vi "b-field one sensor.vi"(0 "magnet location params":T1, 5 "x sensor":dbl, 6 "y sensor":dbl, 7 "z sensor":dbl) -> (20 "Bx (uT)":dbl, 21 "By (uT)":dbl, 22 "Bz (uT)":dbl, 25 "dBx":dbl[](array[numeric]), 26 "dBy":dbl[](array[numeric]), 27 "dBz":dbl[](array[numeric]))   [LabVIEW 2017]
uses:
  typedefs/magnet location fit result.ctl
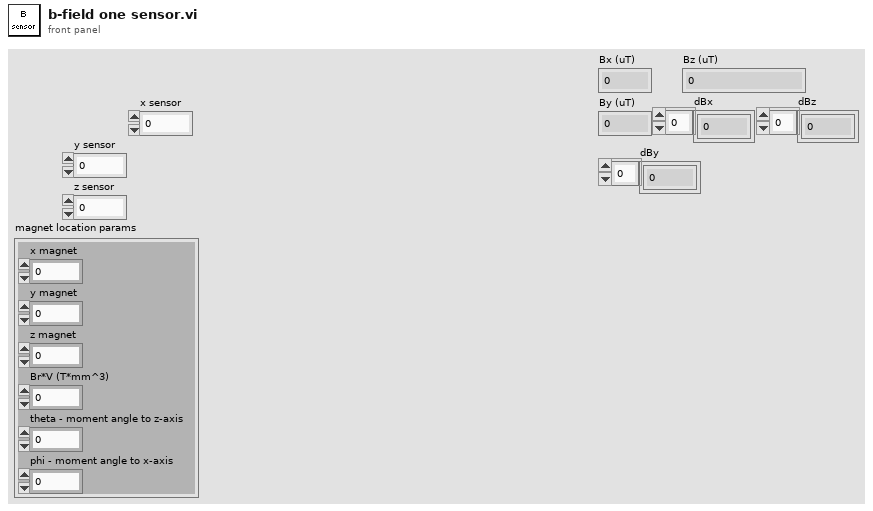
[diagram p1: front panel]
types:
  T1 = typedef "magnet location fit result.ctl" = cluster{"x magnet":dbl, "y magnet":dbl, "z magnet":dbl, "Br*V (T*mm^3)":dbl, "theta - moment angle to z-axis":dbl, "phi - moment angle to x-axis":dbl}
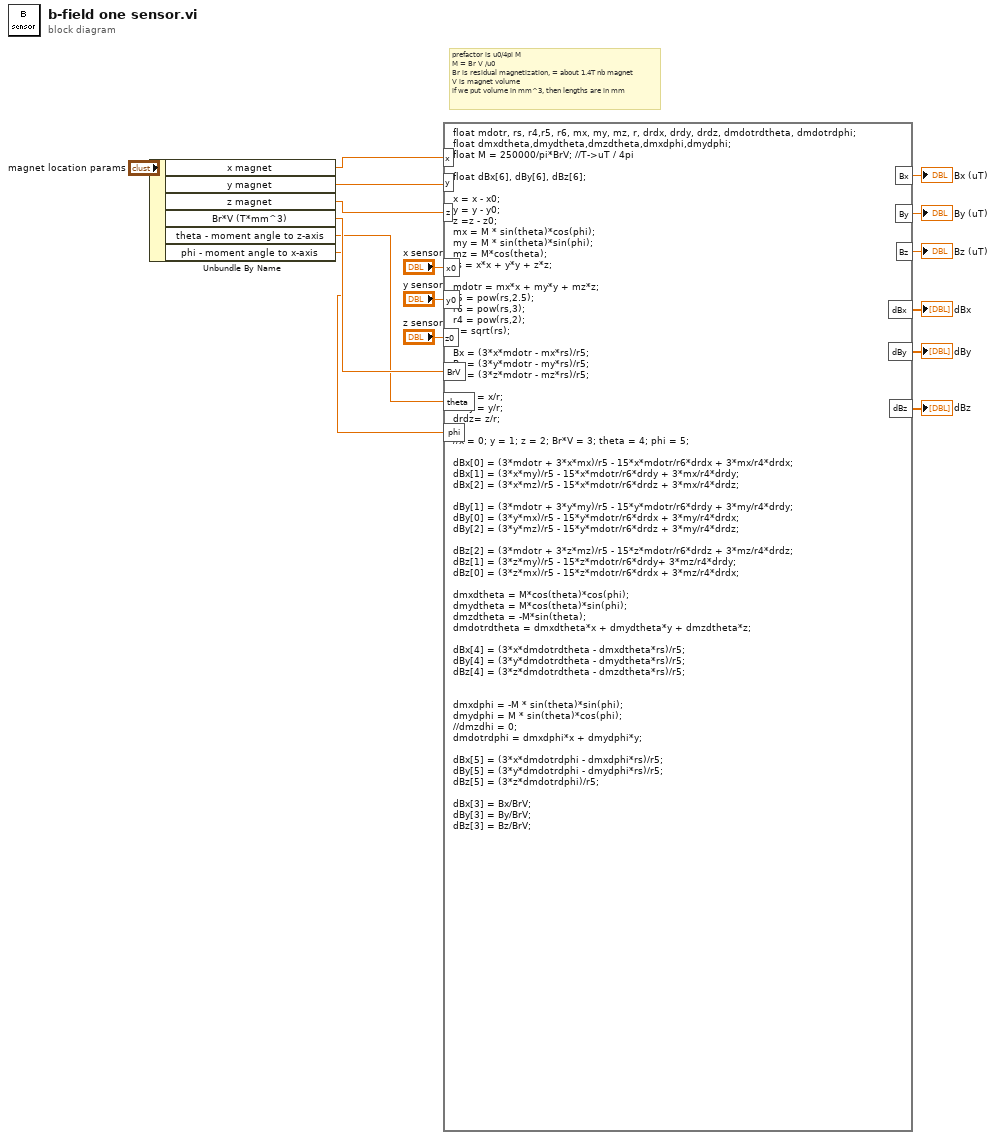
[diagram p0: block diagram]
diagram:
  # "prefactor is u0/4pi M\nM = Br V /u0\nBr is residual magnetization, = about 1.4T nb magnet\nV is magnet volume\nif we put volume in mm^3, then lengths are in mm"
  n1 = Unbundle By Name("magnet location params") -> ("x magnet"=w6:dbl, "y magnet"=w5:dbl, "z magnet"=w4:dbl, "Br*V (T*mm^3)"=w3:dbl, "theta - moment angle to z-axis"=w2:dbl, "phi - moment angle to x-axis"=w1:dbl)
  n2 = formula code="float mdotr, rs, r4,r5, r6, mx, my, mz, r, drdx, drdy, drdz, dmdotrdtheta, dmdotrdphi;\nfloat dmxdtheta,dmydtheta,dmzdtheta,dmxdphi,dmydphi;\nfloat M = 250000/pi*BrV; //T->uT / 4pi\n\nfloat dBx[6], dBy[6], dBz[6];\n\nx = x - x0;\ny = y - y0;\nz =z - z0;\nmx = M * sin(theta)*cos(phi);\nmy = M * sin(theta)*sin(phi);\nmz = M*cos(theta);\nrs = x*x + y*y + z*z;\n\nmdotr = mx*x + my*y + mz*z;\nr5 = pow(rs,2.5);\nr6 = pow(rs,3);\nr4 = pow(rs,2);\nr = sqrt(rs);\n\nBx = (3*x*mdotr - mx*rs)/r5;\nBy = (3*y*mdotr - my*rs)/r5;\nBz = (3*z*mdotr - mz*rs)/r5;\n\ndrdx = x/r;\ndrdy = y/r;\ndrdz= z/r;\n\n//x = 0; y = 1; z = 2; Br*V = 3; theta = 4; phi = 5;\n\ndBx[0] = (3*mdotr + 3*x*mx)/r5 - 15*x*mdotr/r6*drdx + 3*mx/r4*drdx;\ndBx[1] = (3*x*my)/r5 - 15*x*mdotr/r6*drdy + 3*mx/r4*drdy;\ndBx[2] = (3*x*mz)/r5 - 15*x*mdotr/r6*drdz + 3*mx/r4*drdz;\n\ndBy[1] = (3*mdotr + 3*y*my)/r5 - 15*y*mdotr/r6*drdy + 3*my/r4*drdy;\ndBy[0] = (3*y*mx)/r5 - 15*y*mdotr/r6*drdx + 3*my/r4*drdx;\ndBy[2] = (3*y*mz)/r5 - 15*y*mdotr/r6*drdz + 3*my/r4*drdz;\n\ndBz[2] = (3*mdotr + 3*z*mz)/r5 - 15*z*mdotr/r6*drdz + 3*mz/r4*drdz;\ndBz[1] = (3*z*my)/r5 - 15*z*mdotr/r6*drdy+ 3*mz/r4*drdy;\ndBz[0] = (3*z*mx)/r5 - 15*z*mdotr/r6*drdx + 3*mz/r4*drdx;\n\ndmxdtheta = M*cos(theta)*cos(phi);\ndmydtheta = M*cos(theta)*sin(phi);\ndmzdtheta = -M*sin(theta);\ndmdotrdtheta = dmxdtheta*x + dmydtheta*y + dmzdtheta*z;\n\ndBx[4] = (3*x*dmdotrdtheta - dmxdtheta*rs)/r5;\ndBy[4] = (3*y*dmdotrdtheta - dmydtheta*rs)/r5;\ndBz[4] = (3*z*dmdotrdtheta - dmzdtheta*rs)/r5;\n\n\ndmxdphi = -M * sin(theta)*sin(phi);\ndmydphi = M * sin(theta)*cos(phi);\n//dmzdhi = 0;\ndmdotrdphi = dmxdphi*x + dmydphi*y;\n\ndBx[5] = (3*x*dmdotrdphi - dmxdphi*rs)/r5;\ndBy[5] = (3*y*dmdotrdphi - dmydphi*rs)/r5;\ndBz[5] = (3*z*dmdotrdphi)/r5;\n\ndBx[3] = Bx/BrV;\ndBy[3] = By/BrV;\ndBz[3] = Bz/BrV;"("x"=w6, "y"=w5, "z"=w4, "x0"="x sensor", "y0"="y sensor", "z0"="z sensor", "BrV"=w3, "theta"=w2, "phi"=w1) -> ("Bx"=→"Bx (uT)":dbl, "By"=→"By (uT)":dbl, "Bz"=→"Bz (uT)":dbl, "dBx"=→"dBx":dbl[], "dBy"=→"dBy":dbl[], "dBz"=→"dBz":dbl[])
